vi "OCR Get Money2.vi"(7 "error in":errorcluster, 10 "Path":path=path "C:/PokerSS/SS.png") -> (0 "error out":errorcluster, 3 "Player Money":string[](array[string]))   [LabVIEW 2015]
uses:
  <vilib>/vision/NI_Vision_Development_Module.lvlib
panel:
  in  "Parameters":T1={"Threshold Data"={"Method"=enum."Uniform", "Looking for"=1, "Color Mode"=0, "Kernel Size"={"Width"=32, "Height"=32}, "Ranges"=[{"Min"=1, "Max"=255}]}, "Reject Border"=TRUE, "Number Of Erosions"=0, "Size & Spacing"={"Segment Algorithm"=0, "Min Bounding Rect Width"=2, "Max Bounding Rect Width"=7, "Min Bounding Rect Height"=2, "Max Bounding Rect Height"=65536, "Min Character Size"=4, "Max Character Size"=5555, "Min Char Spacing"=1, "Max Horiz Element Spacing"=1, "Max Vert Element Spacing"=0, "Max Space Distance"=65536}, "Read Options"={"Read Strategy"=1, "Read Resolution"=2, "Scale Dependant"=FALSE, "Aspect Ratio"=400, "Acceptance Level"=700, "Substitution Character"="?", "MultiLine"=FALSE}, "Valid Characters"=[], "Use Text Pattern"=FALSE, "Orientation"=0, "# Lines Expected"=0, "Number of Blocks"=4} {"Threshold Data"."Looking for" items=["Light on Dark", "Dark on Light"]; "Threshold Data"."Color Mode" items=["RGB", "HSL", "HSV", "HSI"]; "Size & Spacing"."Segment Algorithm" items=["None", "Shortest Segment", "Legacy Auto Split"]; "Read Options"."Read Strategy" items=["Aggressive", "Conservative"]; "Read Options"."Read Resolution" items=["Low", "Medium", "High"]; "Valid Characters"."Pre-defined characters" items=["Any Character", "User-defined Characters", "Alphabetic", "Alphanumeric", "Uppercase Letters", "Lowercase Letters", "Decimal Digits", "Hexadecimal Digits", "Pattern", "Force Space"]; "Orientation" items=["Baseline inside", "Baseline outside"]}
  in  "All Players Money ROI":T2(array[cluster])=[{"Global Rectangle"=[1068, 495, 1179, 514], "Contours"=[{"ID"=enum."External", "Type"=3, "Coordinates"=[1068, 495, 1179, 514]}]}, {"Global Rectangle"=[1253, 534, 1367, 552], "Contours"=[{"ID"=enum."External", "Type"=3, "Coordinates"=[1253, 534, 1367, 552]}]}, {"Global Rectangle"=[1385, 697, 1502, 712], "Contours"=[{"ID"=enum."External", "Type"=3, "Coordinates"=[1385, 697, 1502, 712]}]}, {"Global Rectangle"=[1264, 838, 1374, 853], "Contours"=[{"ID"=enum."External", "Type"=3, "Coordinates"=[1264, 838, 1374, 853]}]}, {"Global Rectangle"=[1029, 868, 1143, 884], "Contours"=[{"ID"=enum."External", "Type"=3, "Coordinates"=[1029, 868, 1143, 884]}]}, {"Global Rectangle"=[757, 870, 877, 885], "Contours"=[{"ID"=enum."External", "Type"=3, "Coordinates"=[757, 870, 877, 885]}]}, {"Global Rectangle"=[543, 836, 661, 852], "Contours"=[{"ID"=enum."External", "Type"=3, "Coordinates"=[543, 836, 661, 852]}]}, {"Global Rectangle"=[386, 689, 502, 706], "Contours"=[{"ID"=enum."External", "Type"=3, "Coordinates"=[386, 689, 502, 706]}]}, {"Global Rectangle"=[523, 533, 645, 550], "Contours"=[{"ID"=enum."External", "Type"=3, "Coordinates"=[523, 533, 645, 550]}]}, {"Global Rectangle"=[720, 494, 833, 510], "Contours"=[{"ID"=enum."External", "Type"=3, "Coordinates"=[720, 494, 833, 510]}]}]
  out "Image Out":T3(plugin-control)
  out "String (Player1 Money)":string
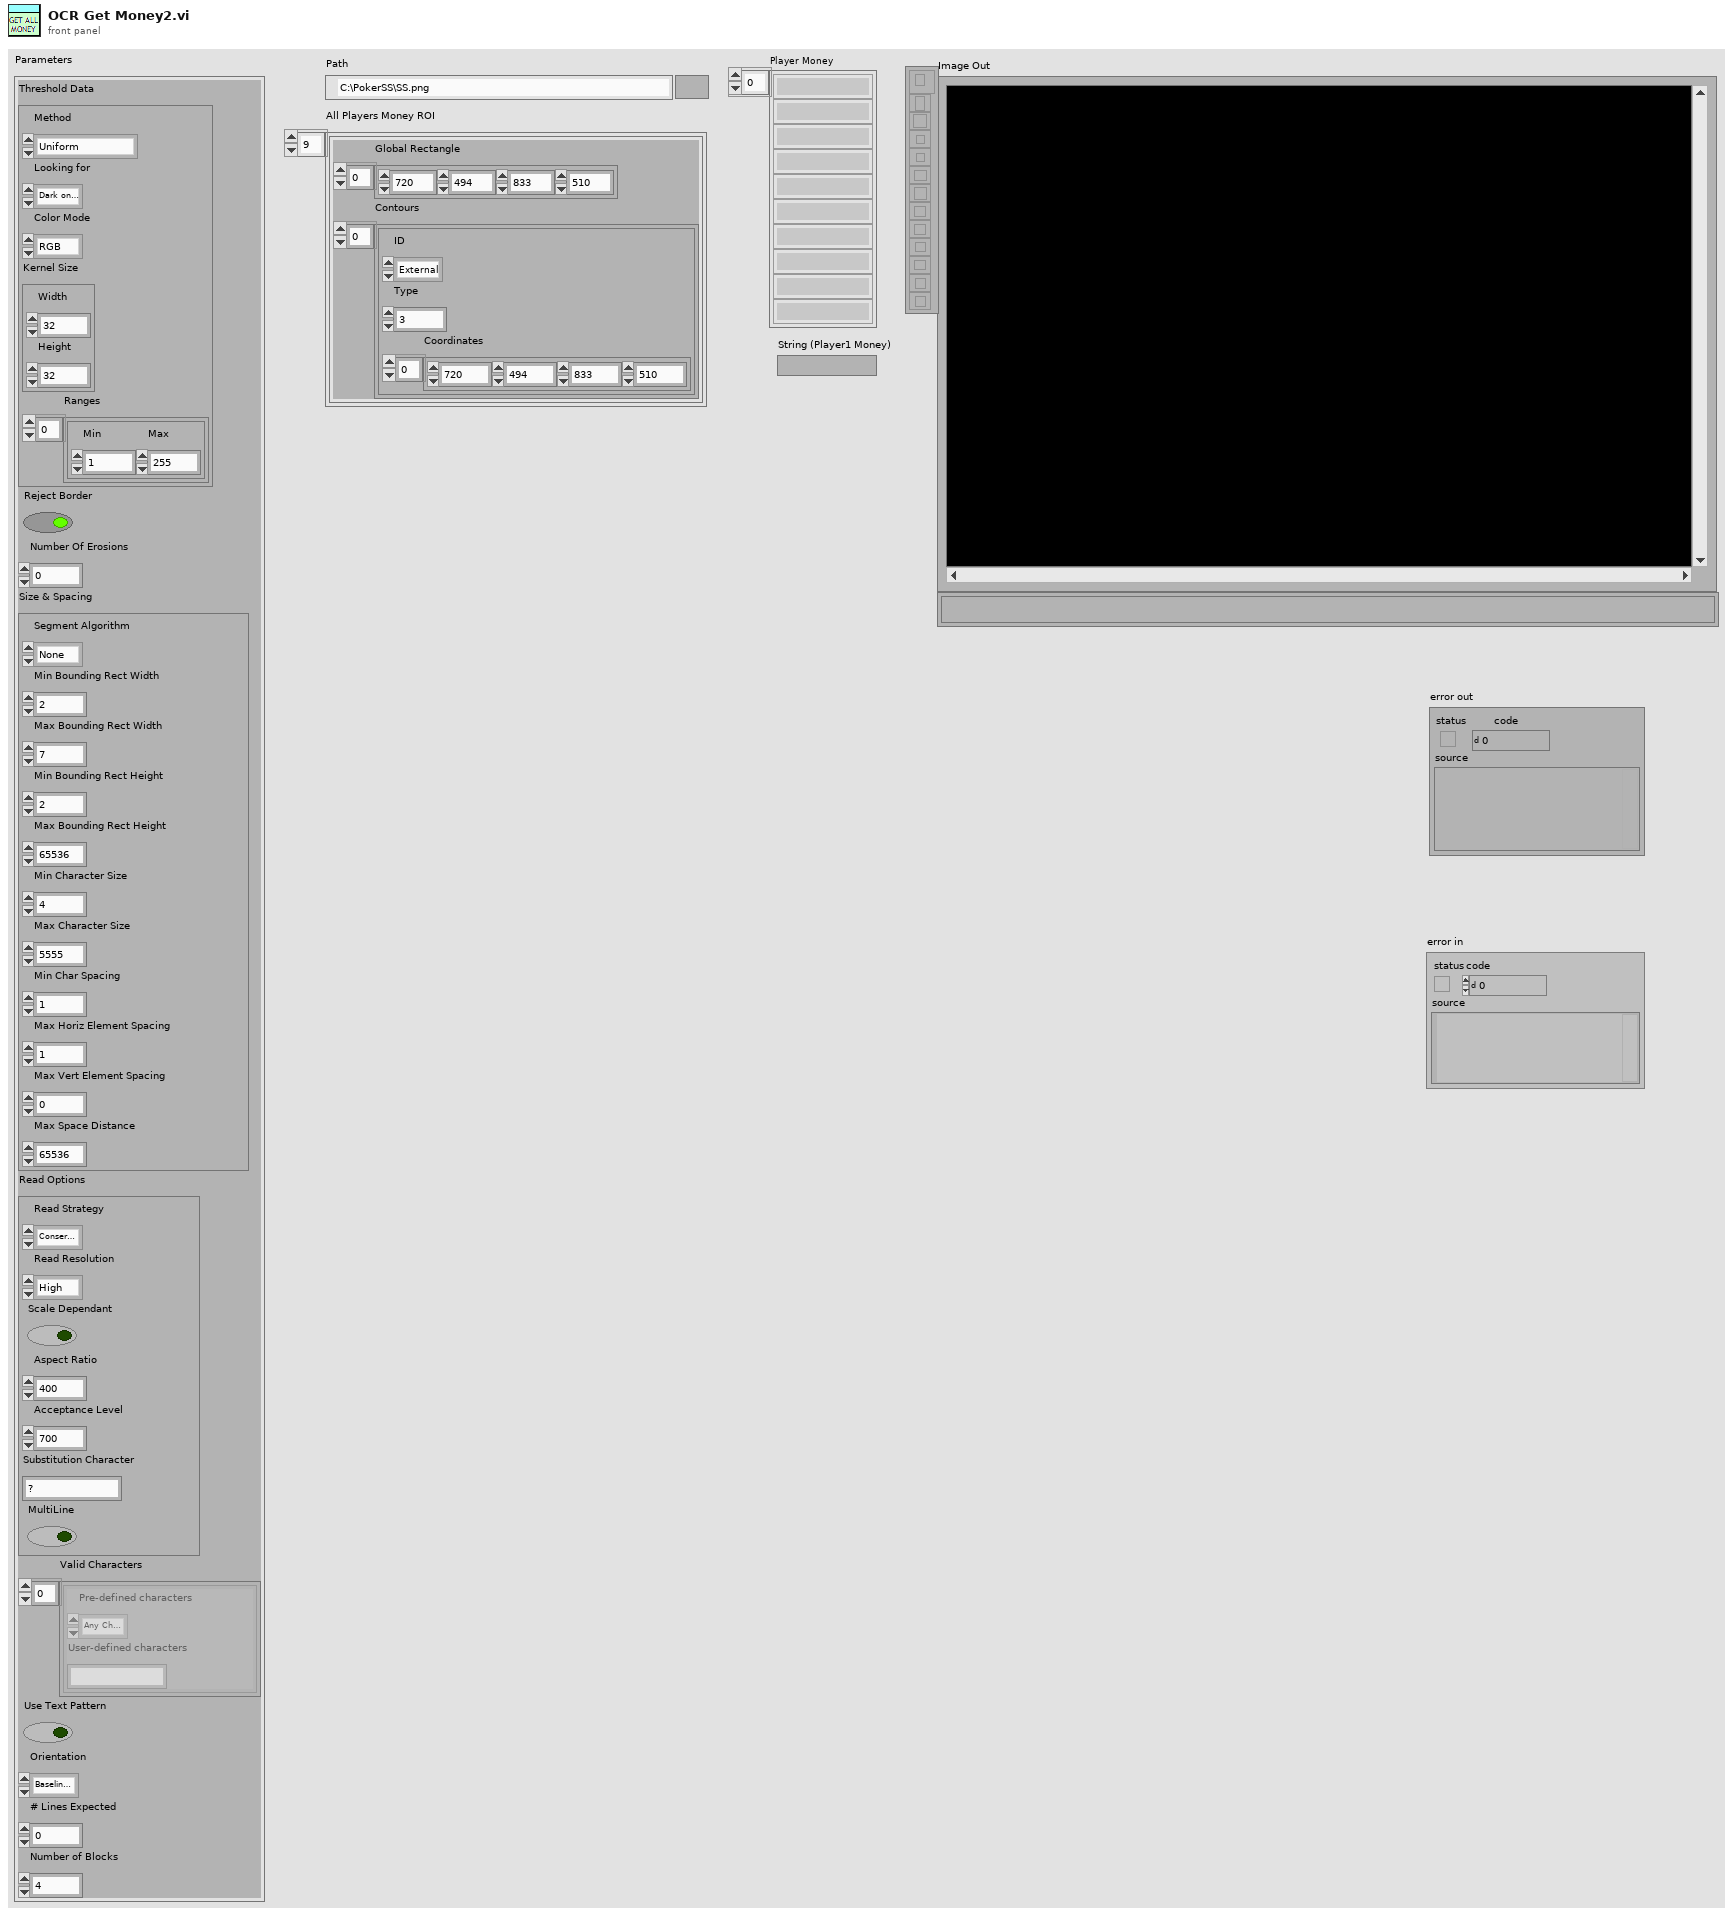
[diagram p1: front panel]
types:
  T1 = cluster{"Threshold Data":cluster{"Method":enum16{"Fixed Range", "Uniform", "Linear", "Non Linear", "Local", "Color"}, "Looking for":u32, "Color Mode":u32, "Kernel Size":cluster{"Width":i32, "Height":i32}, "Ranges":cluster{"Min":i32, "Max":i32}[]}, "Reject Border":bool, "Number Of Erosions":i32, "Size & Spacing":cluster{"Segment Algorithm":u16, "Min Bounding Rect Width":i32, "Max Bounding Rect Width":i32, "Min Bounding Rect Height":i32, "Max Bounding Rect Height":i32, "Min Character Size":i32, "Max Character Size":i32, "Min Char Spacing":i32, "Max Horiz Element Spacing":i32, "Max Vert Element Spacing":i32, "Max Space Distance":i32}, "Read Options":cluster{"Read Strategy":i32, "Read Resolution":i32, "Scale Dependant":bool, "Aspect Ratio":i32, "Acceptance Level":i32, "Substitution Character":string, "MultiLine":bool}, "Valid Characters":cluster{"Pre-defined characters":i32, "User-defined characters":string}[], "Use Text Pattern":bool, "Orientation":u32, "# Lines Expected":u32, "Number of Blocks":i32}
  T2 = cluster{"Global Rectangle":i32[], "Contours":cluster{"ID":enum32{"External", "Internal"}, "Type":u32, "Coordinates":i32[]}[]}[]
  T3 = typedef "IMAQ Image.ctl" = refnum<image>
  T4 = typedef "Image Type" = u32
  T5 = typedef "IMAQ OCR Session.ctl" = refnum<k1>
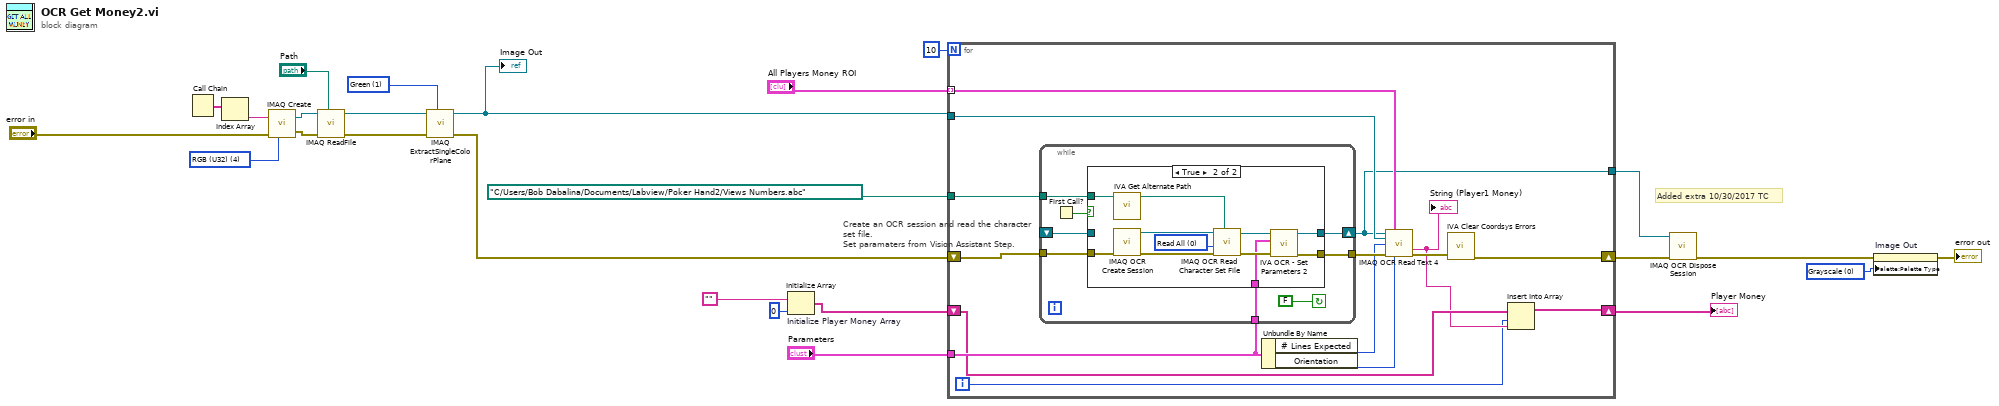
[diagram p0: block diagram]
diagram:
  w12 = u32 0 items=["Grayscale", "Binary", "Gradient", "Rainbow", "Temperature", "User Defined", "Binary 16 Bit", "Gradient 16 Bit", "Rainbow 16 Bit", "Temperature 16 Bit", "User Defined 16 Bit"] ("Palette Type")
  w18 = 1 items=["Red", "Green", "Blue", "Hue", "Saturation", "Luminance", "Value", "Intensity"] ("Color Plane")
  w19 = T4 4 items=["Grayscale (U8)", "Grayscale (I16)", "Grayscale (SGL)", "Complex (CSG)", "RGB (U32)", "HSL (U32)", "RGB (U64)", "Grayscale (U16)"] ("Image Type")
  # "Added extra 10/30/2017 TC"
  n1 = Call Chain() -> (call chain=w21:string[])
  n2 = Index Array(array=w21) -> (element=w20:string)  [unwired: 1 in]
  n3 = call "IMAQ Create"("Image Name"=w20, "Image Type"=w19, "error in (no error)"="error in") -> ("New Image"=w24:T3, "error out"=w23:errorcluster)  [unwired: 1 in, 1 out]
  n4 = call "IMAQ ReadFile"("File Path"="Path", "error in (no error)"=w23, "Image"=w24) -> ("error out"=w25:errorcluster, "Image Out"=w17:T3)  [unwired: 2 in, 5 out]
  n5 = call "IMAQ ExtractSingleColorPlane"("Color Plane"=w18, "error in (no error)"=w25, "Image Src"=w17) -> ("error out"=w16:errorcluster, "Image Dst Out"=w13:T3)  [unwired: 1 in, 6 out]
  "Image Out" <- w13
  n6 = Initialize Array "Initialize Player Money Array"("", 0 ("dimension size")) -> (w7:string[])
  n7 = for {
    N: 10 -> [_]
    tunnel: w13 -> [w33]
    tunnel: path "C:/Users/Bob Dabalina/Documents/Labview/Poker Hand2/Views Numbers.abc" ("File Path") -> [w32]
    tunnel: "All Players Money ROI" -> [w31] mode=indexing
    shift-right: [w34] -> w3
    shift-left: w16 -> [w40]
    tunnel: "Parameters" -> [w39]
    shift-right: [w28] -> w5
    shift-left: w7 -> [w30]
    tunnel: [w26] -> w1
    i -> [w27]
    n8 = while "Create an OCR session and read the character set file.\nSet paramaters from Vision Assistant Step." {
      shift-right: [w45] -> w26
      shift-left: _ -> [w44]
      tunnel: w40 -> [w47]
      tunnel: w39 -> [w43]
      tunnel: w32 -> [w42]
      tunnel: [w41] -> w38
      stop <- FALSE continue-if-true
      n9 = First Call?() -> (First Call?: T/F=w46:bool)
      n10 = case shown="True" w46 {
        tunnel: w42 -> [_ w54]
        tunnel: w47 -> [w49 w58]
        tunnel: [w50 w56] -> w45
        tunnel: [w49 w55] -> w41
        tunnel: w43 -> [_ w51]
        tunnel: w44 -> [w50 _]
        frame False {
        }
        frame True {
          w59 = 0 items=["Read All", "Read Character Set Only", "Read Properties Only"] ("Read Options")
          n11 = call <vilib>:"IVA Get Alternate Path.vi"("Path In"=w54) -> ("Path Out"=w53:path)  [unwired: 10 out]
          n12 = call "IMAQ OCR Create Session"("error in (no error)"=w58) -> ("error out"=w60:errorcluster, "IMAQ OCR Session"=w61:T5)  [unwired: 9 out]
          n13 = call "IMAQ OCR Read Character Set File"("File Path"=w53, "error in (no error)"=w60, "Read Options"=w59, "IMAQ OCR Session"=w61) -> ("error out"=w57:errorcluster, "IMAQ OCR Session (dup)"=w52:T5)  [unwired: 1 in, 5 out]
          n14 = call <vilib>:"IVA OCR - Set Parameters 2.vi"("error in (no error)"=w57, "Parameters"=w51, "IMAQ OCR Session"=w52) -> ("error out"=w55:errorcluster, "IMAQ OCR Session Out"=w56:T5)  [unwired: 7 in]
        }
      }
    }
    n15 = Unbundle By Name(w39) -> ("# Lines Expected"=w36:u32, "Orientation"=w37:u32)
    n16 = call "IMAQ OCR Read Text 4"("IMAQ OCR Session"=w26, "ROI Descriptor"=w31, "Image"=w33, "Number of Lines Requested"=w36, "error in (no error)"=w38, "Orientation"=w37) -> ("Read String"=w29:string, "error out"=w35:errorcluster)  [unwired: 8 out]
    "String (Player1 Money)" <- w29
    n17 = call <vilib>:"IVA Clear Coordsys Errors.vi"("error in (no error)"=w35) -> ("error out"=w34:errorcluster)  [unwired: 10 in]
    n18 = Insert Into Array "Insert Into Array"(array=w30, index=w27, new element=w29) -> (w28:string[])
  }
  "Player Money" <- w5
  n19 = call "IMAQ OCR Dispose Session"("error in (no error)"=w3, "IMAQ OCR Session"=w1) -> ("error out"=w2:errorcluster)  [unwired: 9 in]
  n20 = property on="Image Out" class="ImageControl"(error in=w2, "Palette:Palette Type"=w12) -> (error out=→"error out":errorcluster)  [unwired: 1 in, 1 out]
